vi "Global 4.vi"() -> ()   [LabVIEW 2020]
panel:
  in  "Mode":string
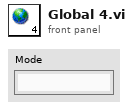
[diagram p1: front panel]
diagram:
